vi "Bind RPC NI_XNET_CAN_Bus_Monitor_API ResetStreamingFilter.vi"(11 "gRPCid server in":T3) -> (0 "error out":errorcluster, 1 "NI_XNET_CAN_Bus_Monitor_API ResetStreamingFilter Internal UE":T2, 2 "NI_XNET_CAN_Bus_Monitor_API ResetStreamingFilter gRPC UE":T1, 3 "gRPCid server out":T3)   [LabVIEW 2025, in "xnet_can_bus_monitor_api_server.lvlib" / "NI_XNET_CAN_Bus_Monitor_API.lvclass"]
uses:
  NI_XNET_CAN_Bus_Monitor_API.lvclass
  <vilib>/gRPC/LabVIEW gRPC Library/Shared/grpcId.ctl
  typeDefs/Server Internal Message UE.ctl
  typeDefs/Server Internal Message.ctl
  <vilib>/gRPC/LabVIEW gRPC Library/Server API/typeDefs/gRPCId Cluster UE.ctl
  <vilib>/gRPC/LabVIEW gRPC Library/Server API/typeDefs/gRPCId Cluster.ctl
  616620f9-6bbe-466a-af51-04bcc3596ea0.vi
  <vilib>/gRPC/LabVIEW gRPC Library/Shared/TranslateGrpcError.vi
  <vilib>/gRPC/LabVIEW gRPC Library/Server API/Server/Get Server DLL Path.vi
  <vilib>/Utility/error.llb/Error Cluster From Error Code.vi
  <vilib>/gRPC/LabVIEW gRPC Library/grpc-lvsupport-release.lvlib
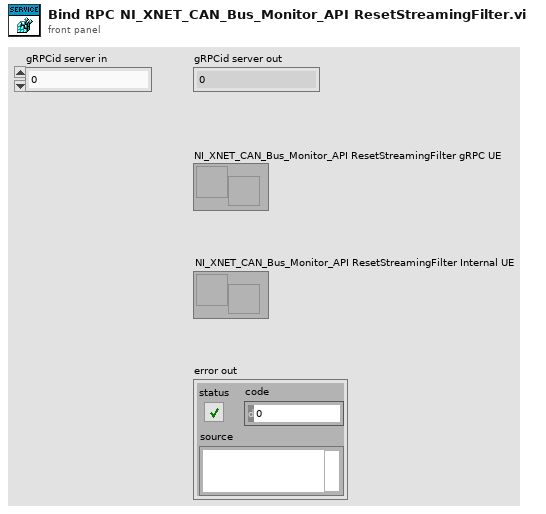
[diagram p1: front panel]
types:
  T1 = typedef "grpc-lvsupport-release.lvlib/gRPCId Cluster UE.ctl" = refnum<user-event>
  T2 = typedef "xnet_can_bus_monitor_api_server.lvlib/NI_XNET_CAN_Bus_Monitor_API.lvclass/Server Internal Message UE.ctl" = refnum<user-event>
  T3 = typedef "grpc-lvsupport-release.lvlib/grpcId.ctl" = u64
  T4 = typedef "xnet_can_bus_monitor_api_server.lvlib/NI_XNET_CAN_Bus_Monitor_API.lvclass/Server Internal Message.ctl" = cluster{"Command":string, "Data":variant}
  T5 = typedef "grpc-lvsupport-release.lvlib/gRPCId Cluster.ctl" = cluster{"gRPCid":T3}
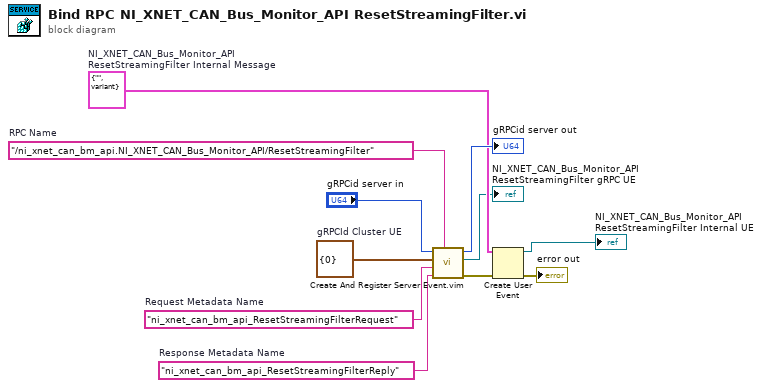
[diagram p0: block diagram]
diagram:
  w5 = T4 {"Command"="", "Data"=variant}  # NI_XNET_CAN_Bus_Monitor_API ResetStreamingFilter Internal Message
  w8 = "ni_xnet_can_bm_api_ResetStreamingFilterReply"  # Response Metadata Name
  w11 = T5 {"gRPCid"=0}  # gRPCId Cluster UE
  w9 = "ni_xnet_can_bm_api_ResetStreamingFilterRequest"  # Request Metadata Name
  w10 = "/ni_xnet_can_bm_api.NI_XNET_CAN_Bus_Monitor_API/ResetStreamingFilter"  # RPC Name
  n1 = call "Create And Register Server Event.vim"("Method name"=w10, "Response Metadata Name"=w8, "Request Metadata Name"=w9, "event in"=w11, "gRPCid server in"="gRPCid server in") -> ("error out"=w4:errorcluster, "event"=→"NI_XNET_CAN_Bus_Monitor_API ResetStreamingFilter gRPC UE":refnum<user-event>, "gRPCid server out"=→"gRPCid server out":T3)  [unwired: 4 in]
  n2 = Create User Event(user event datatype=w5, error in=w4) -> (user event=→"NI_XNET_CAN_Bus_Monitor_API ResetStreamingFilter Internal UE":refnum<user-event>, error out=→"error out":errorcluster)
